vi "Set UDP Settings.vi"(8 "error in (no error)":errorcluster, 10 "Hardware Configuration":T1={"Device Port Number"=2001, "Device IP"="192.168.1.1.100", "Timeout"=5000, "Port Number"=1234}, 11 "Module Configuration":refnum<class "Module Configuration.lvclass">) -> (0 "error out":errorcluster, 3 "Module Configuration out":refnum<class "Module Configuration.lvclass">)   [LabVIEW 2020, in "Plugin.lvlib" / "Plugin_UI.lvclass"]
doc: "Writes hardware settings into module configuration."
uses:
  Plugin_UI.lvclass
  builds/Libraries/LabSys Framework.lvlibp/Configuration Storage/Module Configuration/Module Configuration.lvclass
  UDP Configuration.ctl
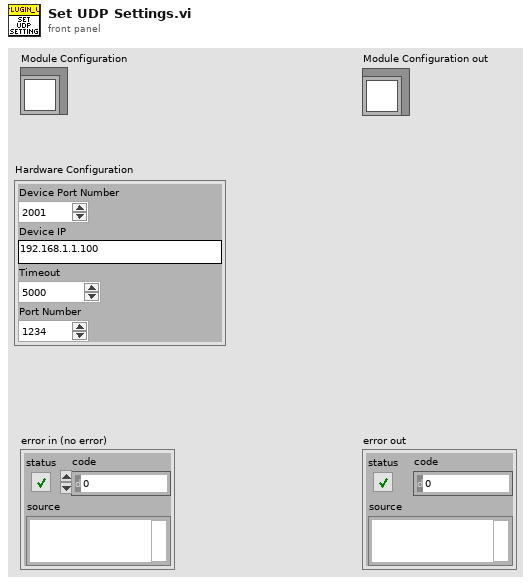
[diagram p1: front panel]
types:
  T1 = typedef "Plugin.lvlib/Plugin_UI.lvclass/UDP Configuration.ctl" = cluster{"Device Port Number":u16, "Device IP":string, "Timeout":i32, "Port Number":u16}
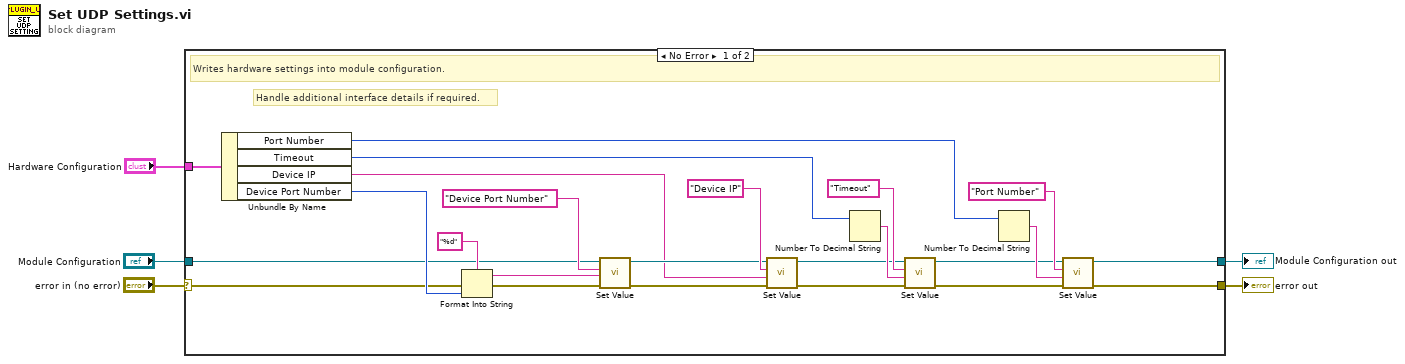
[diagram p0: block diagram]
diagram:
  n1 = case shown="No Error" "error in (no error)" {
    selector: "error in (no error)" -> [w10 w31]
    tunnel: [w6 w31] -> w5
    tunnel: "Module Configuration" -> [w9 w30]
    tunnel: [w7 w30] -> w2
    tunnel: "Hardware Configuration" -> [w8 _]
    frame No Error {
      # "Handle additional interface details if required."
      # "Writes hardware settings into module configuration."
      n2 = Unbundle By Name(w8) -> ("Port Number"=w11:u16, "Timeout"=w12:i32, "Device IP"=w13:string, "Device Port Number"=w14:u16)
      n3 = Format Into String(format string="%d", error in=w10, w14) -> (resulting string=w18:string, error out=w15:errorcluster)  [unwired: 1 in]
      n4 = call "Set Value.vi"("error in (no error)"=w15, "Value"=w18, "Key"="Device Port Number", "Module Configuration in"=w9) -> ("error out"=w19:errorcluster, "Module Configuration out"=w20:refnum<class "Module Configuration.lvclass">)  [unwired: 6 in]
      n5 = call "Set Value.vi"("error in (no error)"=w19, "Value"=w13, "Key"="Device IP", "Module Configuration in"=w20) -> ("error out"=w25:errorcluster, "Module Configuration out"=w22:refnum<class "Module Configuration.lvclass">)  [unwired: 6 in]
      n6 = Number To Decimal String(number=w12) -> (decimal integer string=w28:string)  [unwired: 1 in]
      n7 = call "Set Value.vi"("error in (no error)"=w25, "Value"=w28, "Key"="Timeout", "Module Configuration in"=w22) -> ("error out"=w24:errorcluster, "Module Configuration out"=w23:refnum<class "Module Configuration.lvclass">)  [unwired: 6 in]
      n8 = Number To Decimal String(number=w11) -> (decimal integer string=w27:string)  [unwired: 1 in]
      n9 = call "Set Value.vi"("error in (no error)"=w24, "Value"=w27, "Key"="Port Number", "Module Configuration in"=w23) -> ("error out"=w6:errorcluster, "Module Configuration out"=w7:refnum<class "Module Configuration.lvclass">)  [unwired: 6 in]
    }
    frame Error {
    }
  }
  "error out" <- w5
  "Module Configuration out" <- w2
